vi "DataLog Mirror_srv.vi"(0 "method":T2, 5 "log index":dbl, 7 "certificate":string, 9 "amount":i32, 11 "tag":string, 12 "database":string) -> (4 "size":dbl, 6 "start time":dbl, 8 "points":T1[](array[typedef]) {"value" format="%.3e"; "time" format="%<%H:%M:%S%2u\n%Y/%m/%d>T"}, 10 "string data":string, 15 "error out":errorcluster)   [LabVIEW 2012]
uses:
  typedefs/t_DataLog Mirror Served Methods.ctl
  typedefs/clusters/t_DataLog Point.ctl
  clientsrv/typedefs/t_ClientSrv Access Levels.ctl
  subvis/private/glb_DataLog MCVD.vi
panel:
  # "Update panel typedef\nafter changing panel."
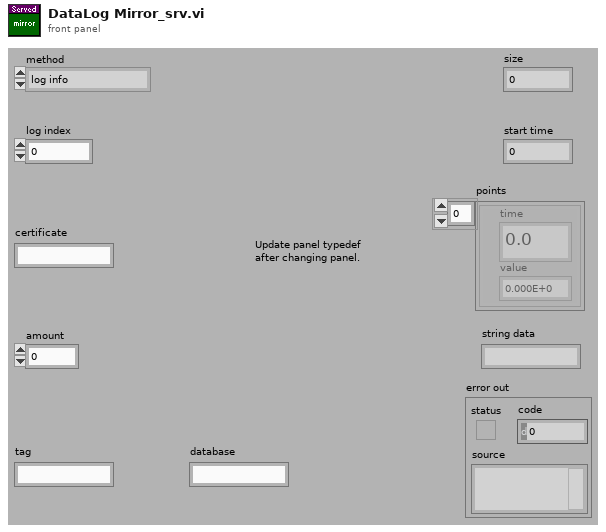
[diagram p1: front panel]
types:
  T1 = typedef "t_DataLog Point.ctl" = cluster{"time":dbl, "value":dbl}
  T2 = typedef "t_DataLog Mirror Served Methods.ctl" = enum16{"log info", "read range", "strsize", "read str"}
  T3 = typedef "t_ClientSrv Access Levels.ctl" = enum16{"observer", "operator", "local"}
  T4 = enum16{"deny read/write", "deny write-only", "deny none"}
  T5 = enum16{"read/write", "read-only", "write-only", "write-only (truncate)"}
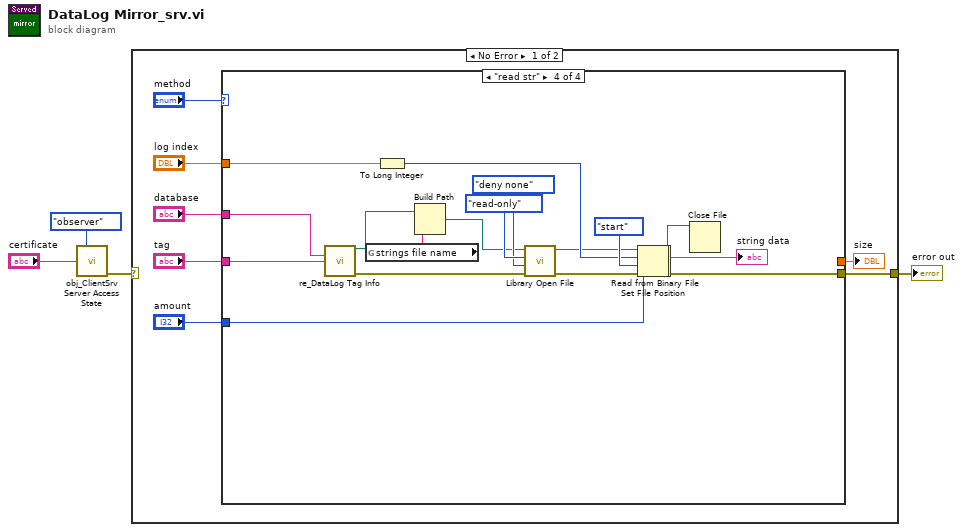
[diagram p0: block diagram]
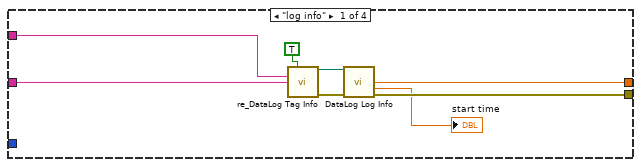
[diagram p2: hidden frame]
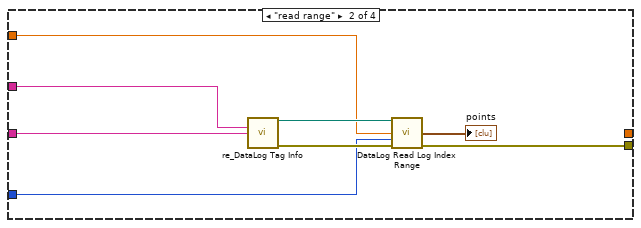
[diagram p3: hidden frame]
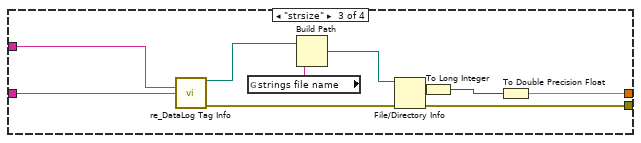
[diagram p4: hidden frame]
diagram:
  n1 = call "obj_ClientSrv Server Access State.vi"("access level"=t_ClientSrv_Access_Levels."observer", "certificate in"="certificate") -> ("error out"=w1:errorcluster)  [unwired: 11 in, 2 out]
  n2 = case shown="No Error" w1 {
    selector: w1 -> [_ w57]
    tunnel: [w11 w57] -> w2
    frame No Error {
      n3 = case shown="\"read str\"" "method" {
        tunnel: "tag" -> [w17 w26 w36 w55]
        tunnel: [w14 w22 w32 w46] -> w11
        tunnel: "database" -> [w18 w27 w37 w56]
        tunnel: "amount" -> [_ w21 _ w47]
        tunnel: [w13 _ w29 _] -> w6
        tunnel: "log index" -> [_ w20 _ w48]
        frame "log info" {
          n4 = call "re_DataLog Tag Info.vi"("flush? (false)"=TRUE, "database (current)"=w18, "tag"=w17) -> ("tag log directory"=w15:path, "error out"=w16:errorcluster)  [unwired: 9 in, 2 out]
          n5 = call "DataLog Log Info.vi"("tag log directory"=w15, "error in (no error)"=w16) -> ("size"=w13:dbl, "start time"=→"start time":dbl, "error out"=w14:errorcluster)  [unwired: 10 in, 1 out]
        }
        frame "read range" {
          n6 = call "re_DataLog Tag Info.vi"("database (current)"=w27, "tag"=w26) -> ("tag log directory"=w25:path, "error out"=w24:errorcluster)  [unwired: 10 in, 2 out]
          n7 = call "DataLog Read Log Index Range.vi"("tag log directory"=w25, "log index"=w20, "number of points"=w21, "error in (no error)"=w24) -> ("range of points"=→"points":T1[], "error out"=w22:errorcluster)  [unwired: 9 in, 1 out]
        }
        frame "strsize" {
          n8 = call "re_DataLog Tag Info.vi"("database (current)"=w37, "tag"=w36) -> ("tag log directory"=w34:path, "error out"=w33:errorcluster)  [unwired: 10 in, 2 out]
          n9 = global read "glb_DataLog MCVD.vi" "strings file name"() -> (w35:string)
          n10 = Build Path(base path=w34, name or relative path=w35) -> (appended path=w31:path)
          n11 = File/Directory Info(path=w31, error in=w33) -> (size=w28:i64, error out=w32:errorcluster)  [unwired: 5 out]
          n12 = To Long Integer(number=w28) -> (32bit integer=w30:i32)
          n13 = To Double Precision Float(number=w30) -> (double precision float=w29:dbl)
        }
        frame "read str" {
          n14 = call "re_DataLog Tag Info.vi"("database (current)"=w56, "tag"=w55) -> ("tag log directory"=w53:path, "error out"=w50:errorcluster)  [unwired: 10 in, 2 out]
          n15 = global read "glb_DataLog MCVD.vi" "strings file name"() -> (w54:string)
          n16 = To Long Integer(number=w48) -> (32bit integer=w43:i32)
          n17 = Build Path(base path=w53, name or relative path=w54) -> (appended path=w49:path)
          n18 = call "Library Open File.vi"("error in (no error)"=w50, "deny mode (deny none)"=T4."deny none" ("deny mode (2)"), "open mode (read/write)"=T5."read-only" ("open mode (0)"), "file path"=w49) -> ("error out"=w41:errorcluster, "refnum"=w42:refnum<file>)  [unwired: 2 in]
          n19 = Set File Position(offset (in bytes) (0)=w43, refnum=w42, from (0:start)=enum16{"start", "end", "current"}."start" ("pos mode (0:2)"), error in=w41) -> (refnum out=w39:refnum<file>, error out=w38:errorcluster)
          n20 = Read from Binary File(8:w38, 10:w47, 11:w39) -> (0:w46:errorcluster, 2:→"string data":string, 3:w40:refnum<file>)  [unwired: 3 in, 1 out]
          n21 = Close File(refnum=w40) -> ()  [unwired: 1 in, 2 out]
        }
      }
      "size" <- w6
    }
    frame Error {
    }
  }
  "error out" <- w2
